vi "Save Instrument.vi"(8 "error in (no error)":errorcluster, 11 "CSM-Helper in":refnum<class "CSM-Helper.lvclass">) -> (0 "error out":errorcluster, 3 "CSM-Helper out":refnum<class "CSM-Helper.lvclass">)   [LabVIEW 2017, in "CSM-Helper.lvclass"]
doc: "### Save Instrument.vi\n\n-- <b>Controls</b> --\n- <b>CSM-Helper in</b>: CSMHelper input\n\n-- <b>Indicators</b> --\n- <b>CSM-Helper out</b>: CSMHelper output"
uses:
  CSM-Helper.lvclass
  CSM-Helper.lvclass/CSM-Helper.ctl
  Properties/Read VI Ref.vi
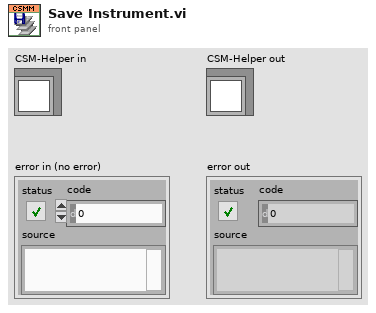
[diagram p1: front panel]
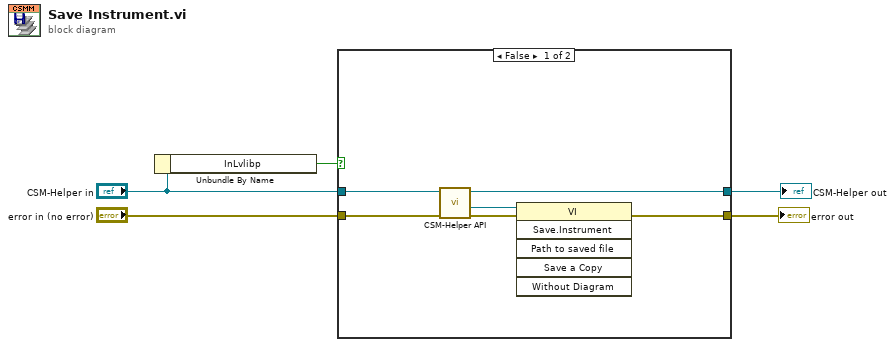
[diagram p0: block diagram]
diagram:
  n1 = Unbundle By Name("CSM-Helper in") -> ("InLvlibp"=w1:bool)
  n2 = case shown="False" w1 {
    tunnel: [w11 w12] -> w5
    tunnel: "error in (no error)" -> [w10 w13]
    tunnel: [w9 w13] -> w3
    tunnel: "CSM-Helper in" -> [w8 w12]
    frame False {
      n3 = call-poly "CSM-Helper API.vi"("error in (no error)"=w10, "CSM-Helper in"=w8) -> ("error out"=w7:errorcluster, "VI"=w6:refnum<vi>, "CSM-Helper out"=w11:refnum<class "CSM-Helper.lvclass">)  [unwired: 7 in]
      n4 = invoke on="Invoke Node" class="VI" method="Save.Instrument"(reference=w6, error in=w7) -> (error out=w9:errorcluster)  [unwired: 4 in, 5 out]
    }
    frame True {
    }
  }
  "CSM-Helper out" <- w5
  "error out" <- w3
